vi "Write SamplesperCycle.vi"(8 "error in (no error)":errorcluster, 10 "SamplesperCycle":u16, 11 "Change Samples per Cycle CMD in":refnum<class "Change Samples per Cycle CMD.lvclass">) -> (0 "error out":errorcluster, 3 "Change Samples per Cycle CMD out":refnum<class "Change Samples per Cycle CMD.lvclass">)   [LabVIEW 2017, in "gCRDS.lvlib" / "Change Samples per Cycle CMD.lvclass"]
uses:
  Change Samples per Cycle CMD.lvclass
  Change Samples per Cycle CMD.lvclass/Change Samples per Cycle CMD.ctl
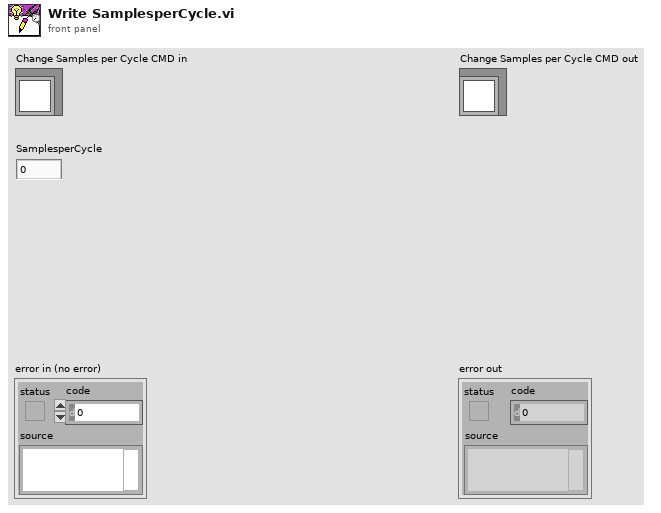
[diagram p1: front panel]
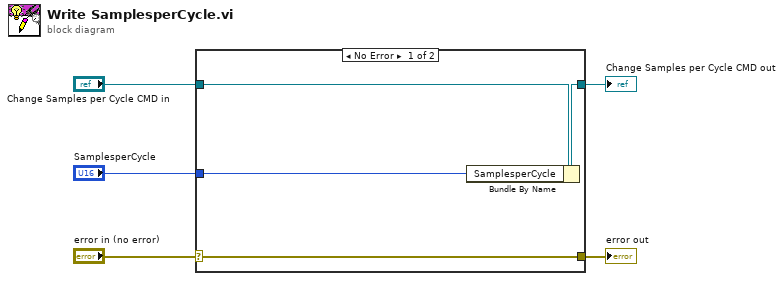
[diagram p0: block diagram]
diagram:
  n1 = case shown="No Error" "error in (no error)" {
    selector: "error in (no error)" -> [w9 w10]
    tunnel: [w9 w10] -> w4
    tunnel: [w7 w11] -> w2
    tunnel: "Change Samples per Cycle CMD in" -> [w8 w11]
    tunnel: "SamplesperCycle" -> [w6 _]
    frame No Error {
      n2 = Bundle By Name(cluster=w8, "SamplesperCycle"=w6) -> (w7:refnum<class "Change Samples per Cycle CMD.lvclass">)
    }
    frame Error {
    }
  }
  "error out" <- w4
  "Change Samples per Cycle CMD out" <- w2
